vi "LS-335_Hardware_Module.vi"(5 "Enable":bool=TRUE, 6 "PID Settings":T2={"Heater Output (1:1)"=1, "Gain (P) (50.0)"=50.0, "Reset (I) (20.0)"=20.0, "Rate (D) (0.0 %)"=0.0, "Range (0:Off)"=0, "Manual Output (0.00 %)"=0.0} {"Heater Output (1:1)" items=["1"=1, "2"=2]; "Range (0:Off)" items=["Off", "Low (On)", "Medium", "High"]; "Manual Output (0.00 %)" format="%.2f"; "Rate (D) (0.0 %)" format="%.1f"; "Reset (I) (20.0)" format="%.1f"; "Gain (P) (50.0)" format="%.1f"}, 7 "Command":T3, 8 "error in (no error)":errorcluster, 9 "Ramp Rate (0.0)":dbl format="%.1f", 10 "Setpoint (0.0000)":dbl format="%.4f", 11 "VISA resource name":refnum<visa-resource-name>="GPIB0::5::INSTR") -> (0 "error out":errorcluster, 1 "Sensor Data":dbl format="%.4f", 2 "Setpoint":dbl format="%.4f", 3 "Output Value":dbl format="%.1f")   [LabVIEW 2017]
uses:
  LS-335_Hardware_Module Control.ctl
  LS-335 SET PID.ctl
  <instrlib>/Lake Shore 335/Public/Data/Sensor Data (Single Reading).vi
  <instrlib>/Lake Shore 335/Lake Shore 335.lvlib
panel:
  out "Heater Output (1:1)":u16(ring)=1 items=["1"=1, "2"=2]
  out "Power Up Enable (F: Off)":bool
  out "Heater Resistance (1:25 Ohm)":u16(ring)=1 items=["25 Ohm"=1, "50 Ohm"=2]
  out "Input (0:None)":u16(ring)=1 items=["None", "A", "B"]
  out "Mode (0:Off)":u16(ring) items=["Off", "Closed Loop PID", "Zone", "Open Loop", "Monitor Out", "Warmup Supply"]
  out "Max Current (0:User Specified)":u16(ring) items=["User Specified", "0.707 A", "1.0 A", "1.141 A", "1.732 A"]
  out "Max User Current (1.732)":dbl=1.732 format="%.3f"
  out "Heater Out Display (1:Current)":u16(ring)=1 items=["Current"=1, "Power"=2]
  out "Polarity (0:Unipolar)":u16(ring) items=["Unipolar", "Bipolar"]
  out "Output Type (0:Current)":u16(ring) items=["Current", "Voltage"]
  out "Data Source (0:Kelvin)":u16(ring) items=["Kelvin", "Celsius", "Sensor Units"]
  out "Input (0:A)":u16(ring) items=["A", "B"]
  in  "Serial Configuration":T1={"Baud Rate"=57600, "Parity"=1, "Data Bits"=7, "Stop Bits"=10, "Flow Control"=0} {"Flow Control" items=["None", "XON/XOFF", "RTS/CTS", "XON/XOFF & RTS/CTS", "DTR/DSR", "XON/XOFF & DTR/DSR"]; "Stop Bits" items=["1.0"=10, "1.5"=15, "2.0"=20]; "Data Bits" items=["7"=7, "8"=8]; "Parity" items=["None", "Odd", "Even", "Mark", "Space"]; "Baud Rate" items=["300"=300, "600"=600, "1200"=1200, "2400"=2400, "4800"=4800, "9600"=9600, "19200"=19200, "38400"=38400, "57600"=57600]}
  # "LAKE SHORE MODEL 335"
  # "INTERNAL VI SETTINGS. No accesibles desde fuera"
  # "Settings for Either Heater Output"
  # "Settings for Heater Output 2 Only"
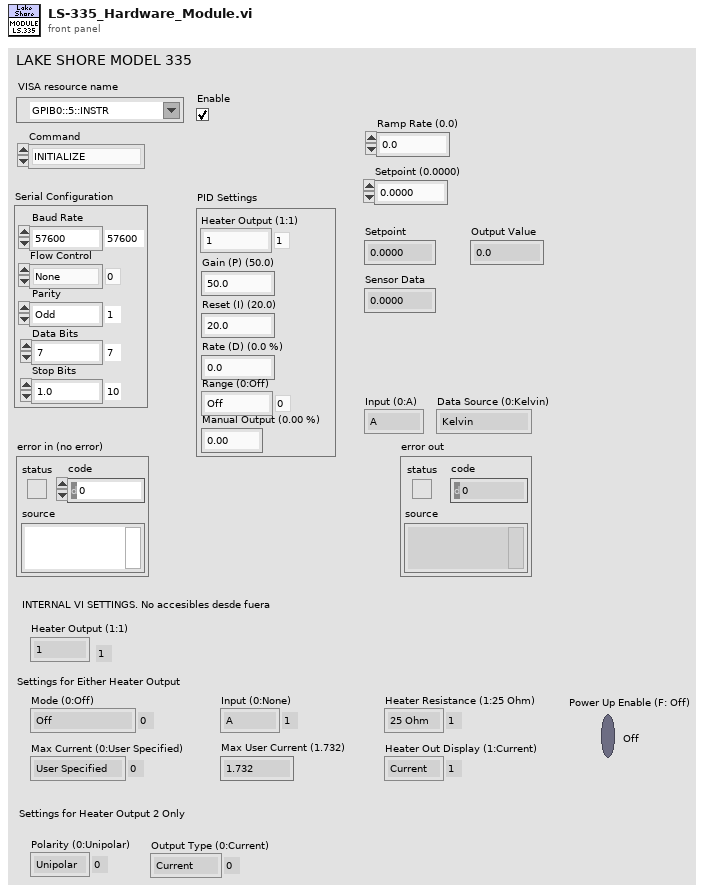
[diagram p1: front panel]
types:
  T1 = cluster{"Baud Rate":u32, "Parity":u16, "Data Bits":u16, "Stop Bits":u16, "Flow Control":u16}
  T2 = typedef "LS-335 SET PID.ctl" = cluster{"Heater Output (1:1)":u16, "Gain (P) (50.0)":dbl, "Reset (I) (20.0)":dbl, "Rate (D) (0.0 %)":dbl, "Range (0:Off)":u16, "Manual Output (0.00 %)":dbl}
  T3 = typedef "LS-335_Hardware_Module Control.ctl" = enum16{"INITIALIZE", "READ TEMPERATURE", "READ CONTROL DATA", "WRITE SETPOINT AND RATE", "WRITE PID AND POWER RANGE", "WRITE CONTROL PARAMETERS", "WRITE INPUT PARAMETERS", "SHUTDOWN"}
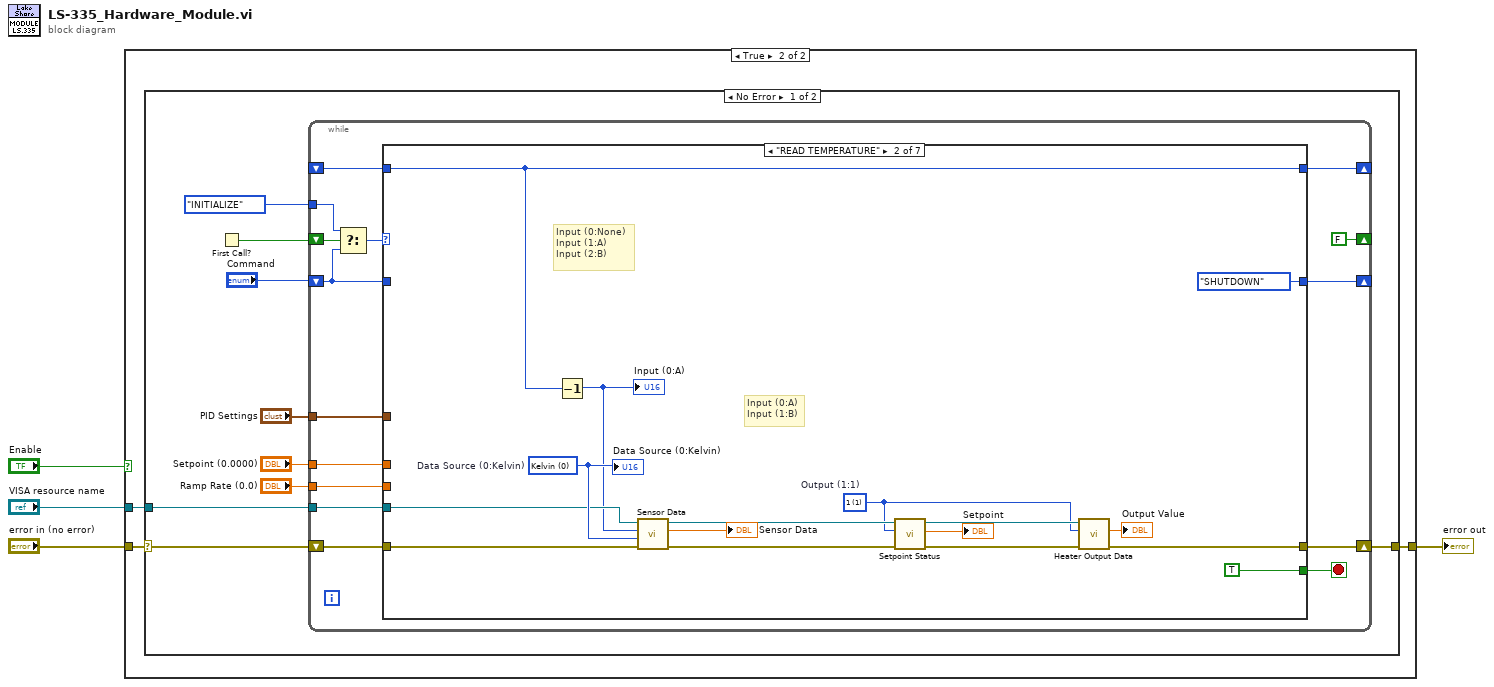
[diagram p0: block diagram]
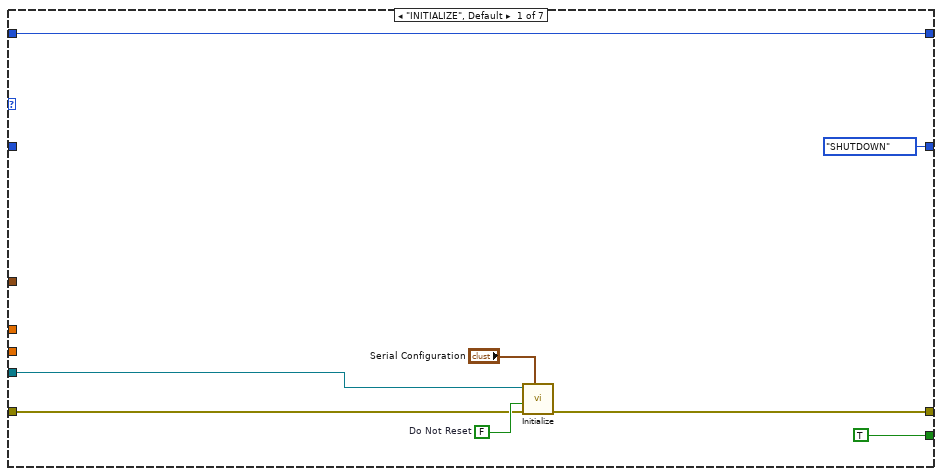
[diagram p3: hidden frame]
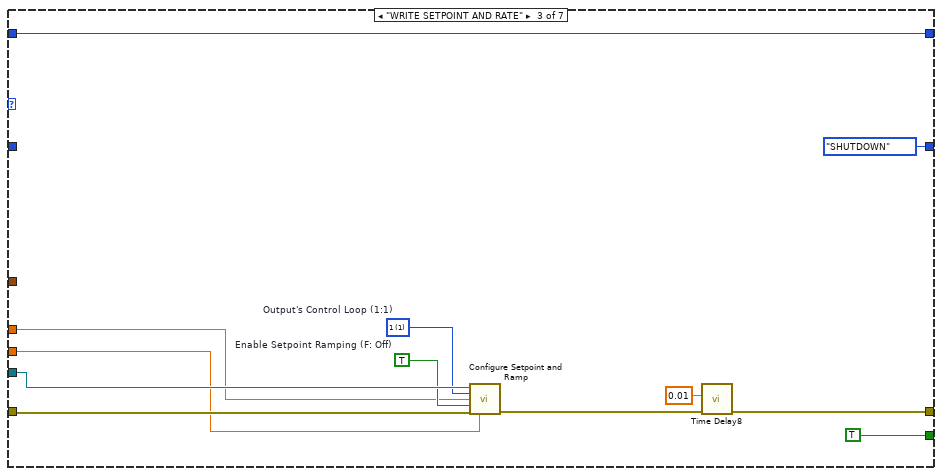
[diagram p4: hidden frame]
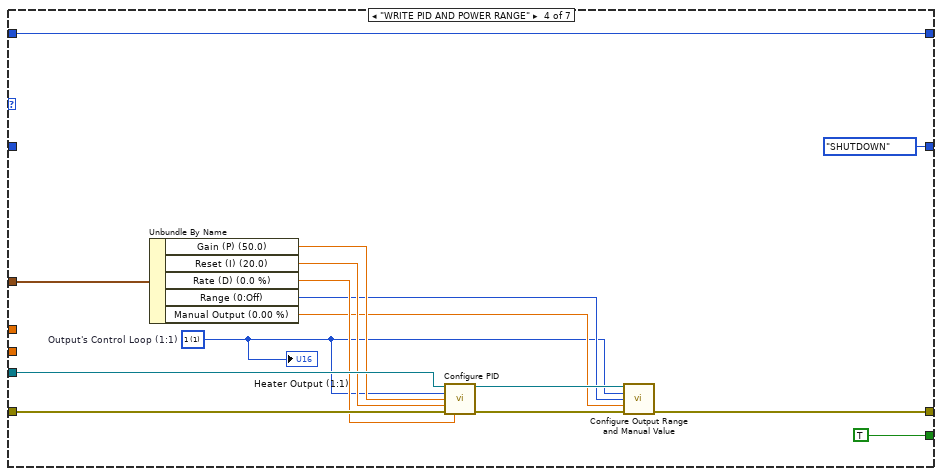
[diagram p5: hidden frame]
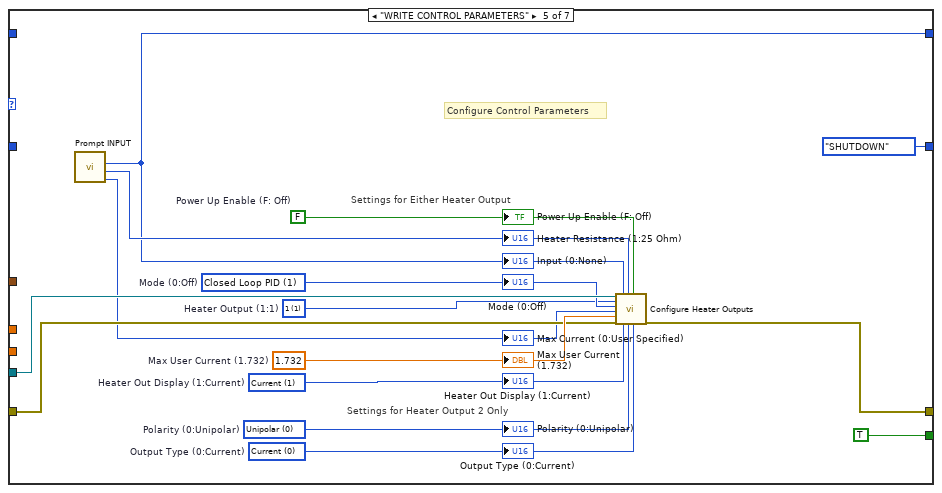
[diagram p6: hidden frame]
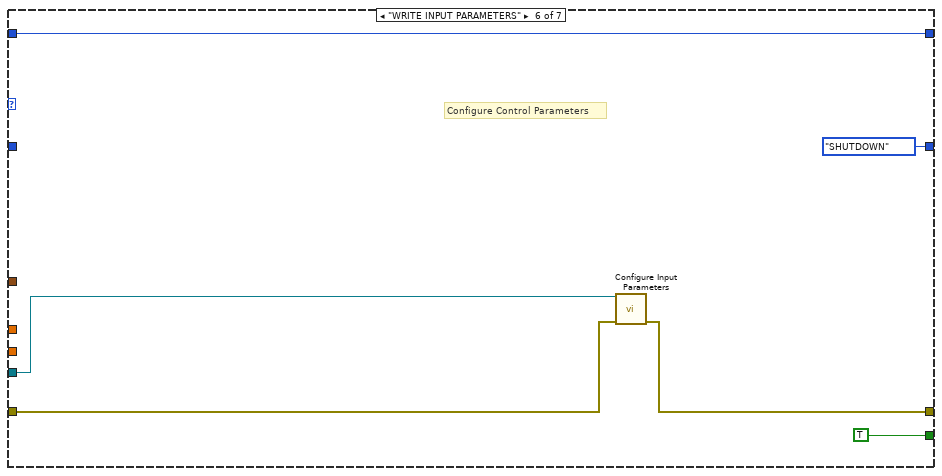
[diagram p7: hidden frame]
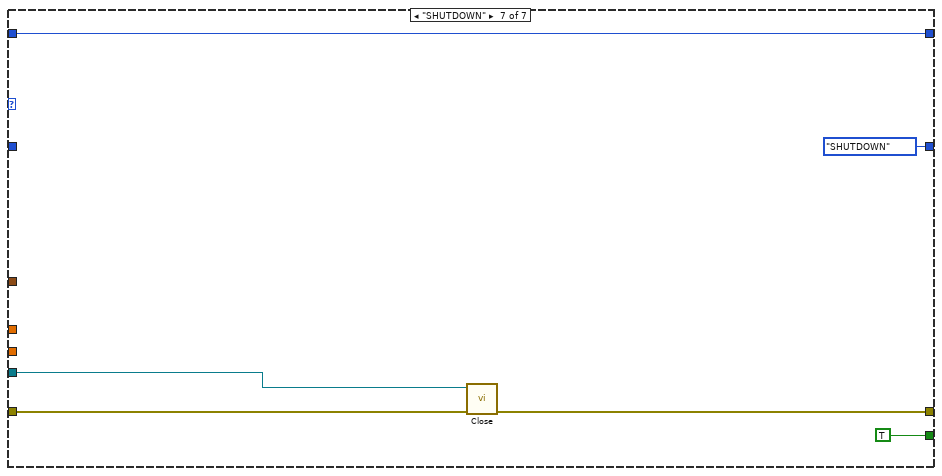
[diagram p8: hidden frame]
diagram:
  n1 = case shown="True" "Enable" {
    tunnel: "error in (no error)" -> [w5 w8]
    tunnel: [w5 w7] -> w3
    tunnel: "VISA resource name" -> [_ w6]
    frame False {
    }
    frame True {
      n2 = case shown="No Error" w8 {
        selector: w8 -> [w15 w111]
        tunnel: [w14 w111] -> w7
        tunnel: w6 -> [w12 _]
        frame No Error {
          n3 = First Call?() -> (First Call?: T/F=w17:bool)
          n4 = while {
            shift-right: [w27] -> _
            shift-left: "Command" -> [w28]
            shift-right: [w25] -> w14
            shift-left: w15 -> [w24]
            shift-right: [FALSE ("First Call?: T/F")] -> _
            shift-left: w17 -> [w32]
            tunnel: LS-335_Hardware_Module_Control."INITIALIZE" ("t") -> [w31]
            tunnel: w12 -> [w23]
            tunnel: "Setpoint (0.0000)" -> [w22]
            tunnel: "Ramp Rate (0.0)" -> [w21]
            tunnel: "PID Settings" -> [w20]
            shift-right: [w19] -> _
            shift-left: _ -> [w18]
            stop <- w26 stop-if-true
            n5 = Select(t=w31, s=w32, f=w28) -> (s? t:f=w29:T3)
            n6 = case shown="\"READ TEMPERATURE\"" w29 {
              tunnel: w28 -> [_ _ _ _ _ _ _]
              tunnel: [LS-335_Hardware_Module_Control."SHUTDOWN" ("s? t:f") LS-335_Hardware_Module_Control."SHUTDOWN" ("s? t:f") LS-335_Hardware_Module_Control."SHUTDOWN" ("s? t:f") LS-335_Hardware_Module_Control."SHUTDOWN" ("s? t:f") LS-335_Hardware_Module_Control."SHUTDOWN" ("s? t:f") LS-335_Hardware_Module_Control."SHUTDOWN" ("s? t:f") LS-335_Hardware_Module_Control."SHUTDOWN" ("s? t:f")] -> w27
              tunnel: [TRUE ("First Call?: T/F") TRUE ("First Call?: T/F") TRUE ("First Call?: T/F") TRUE ("First Call?: T/F") TRUE ("First Call?: T/F") TRUE ("First Call?: T/F") TRUE ("First Call?: T/F")] -> w26
              tunnel: [w36 w44 w66 w75 w90 w103 w108] -> w25
              tunnel: w24 -> [w37 w53 w65 w81 w91 w100 w107]
              tunnel: w23 -> [w35 w54 w63 w82 w92 w101 w109]
              tunnel: w22 -> [_ _ w60 _ _ _ _]
              tunnel: w21 -> [_ _ w59 _ _ _ _]
              tunnel: w20 -> [_ _ _ w71 _ _ _]
              tunnel: [w33 w42 w57 w69 w84 w99 w105] -> w19
              tunnel: w18 -> [w33 w42 w57 w69 _ w99 w105]
              frame "INITIALIZE", Default {
                w38 = FALSE  # Do Not Reset
                n7 = call <instrlib>:"Initialize.vi"("Serial Configuration"="Serial Configuration", "error in (no error)"=w37, "Reset (True)"=w38, "VISA resource name"=w35) -> ("error out"=w36:errorcluster)  [unwired: 6 in, 1 out]
              }
              frame "READ TEMPERATURE" {
                w46 = u16 1 items=["1"=1, "2"=2]  # Output (1:1)
                w55 = u16 0 items=["Kelvin", "Celsius", "Sensor Units"]  # Data Source (0:Kelvin)
                # "Input (0:A)\nInput (1:B)"
                # "Input (0:None)\nInput (1:A)\nInput (2:B)"
                n8 = Decrement(x=w42) -> (x-1=w41:u16)
                "Input (0:A)" <- w41
                n9 = call-poly <instrlib>:"Sensor Data.vi"("error in (no error)"=w53, "Data Source (0:Kelvin)"=w55, "Input (0:A)"=w41, "VISA resource name"=w54) -> ("error out"=w49:errorcluster, "Sensor Data"=→"Sensor Data":dbl, "VISA resource name out"=w50:refnum<visa-resource-name>)  [unwired: 5 in]
                n10 = call <instrlib>:"Setpoint Status.vi"("error in (no error)"=w49, "Output (1:1)"=w46, "VISA resource name"=w50) -> ("error out"=w45:errorcluster, "Setpoint"=→"Setpoint":dbl, "VISA resource name out"=w47:refnum<visa-resource-name>)  [unwired: 6 in]
                n11 = call <instrlib>:"Heater Output Data.vi"("error in (no error)"=w45, "Heater Output (1:1)"=w46, "VISA resource name"=w47) -> ("error out"=w44:errorcluster, "Output Value"=→"Output Value":dbl)  [unwired: 6 in, 1 out]
                "Data Source (0:Kelvin)" <- w55
              }
              frame "WRITE SETPOINT AND RATE" {
                w61 = TRUE  # Enable Setpoint Ramping (F: Off)
                w62 = u16 1 items=["1"=1, "2"=2]  # Output's Control Loop (1:1)
                n12 = call <instrlib>:"Configure Setpoint and Ramp.vi"("VISA resource name"=w63, "Output's Control Loop (1:1)"=w62, "Setpoint (0.0000)"=w60, "Enable Setpoint Ramping (F: Off)"=w61, "error in (no error)"=w65, "Ramp Rate (0.0)"=w59) -> ("error out"=w64:errorcluster)  [unwired: 8 in, 1 out]
                n13 = call "Time Delay8"("error in (no error)"=w64, "Delay Time (s)"=0.01) -> ("error out"=w66:errorcluster)  [unwired: 9 in]
              }
              frame "WRITE PID AND POWER RANGE" {
                w70 = u16 1 items=["1"=1, "2"=2]  # Output's Control Loop (1:1)
                n14 = Unbundle By Name(w71) -> ("Gain (P) (50.0)"=w80:dbl, "Reset (I) (20.0)"=w79:dbl, "Rate (D) (0.0 %)"=w78:dbl, "Range (0:Off)"=w73:u16, "Manual Output (0.00 %)"=w74:dbl)
                n15 = call <instrlib>:"Configure PID.vi"("VISA resource name"=w82, "Output's Control Loop (1:1)"=w70, "Gain (P) (50.0)"=w80, "Reset (I) (20.0)"=w79, "error in (no error)"=w81, "Rate (D) (0.0 %)"=w78) -> ("VISA resource name out"=w77:refnum<visa-resource-name>, "error out"=w76:errorcluster)  [unwired: 8 in]
                n16 = call <instrlib>:"Configure Output Range and Manual Value.vi"("VISA resource name"=w77, "Heater Output (1:1)"=w70, "Range (0:Off)"=w73, "Manual Output (0.00 %)"=w74, "error in (no error)"=w76) -> ("error out"=w75:errorcluster)  [unwired: 9 in, 1 out]
                "Heater Output (1:1)" <- w70
              }
              frame "WRITE CONTROL PARAMETERS" {
                w87 = u16 1 items=["1"=1, "2"=2]  # Heater Output (1:1)
                w94 = 1.732  # Max User Current (1.732)
                w95 = u16 1 items=["Current"=1, "Power"=2]  # Heater Out Display (1:Current)
                w96 = u16 0 items=["Unipolar", "Bipolar"]  # Polarity (0:Unipolar)
                w97 = u16 0 items=["Current", "Voltage"]  # Output Type (0:Current)
                w93 = FALSE  # Power Up Enable (F: Off)
                w88 = u16 1 items=["Off", "Closed Loop PID", "Zone", "Open Loop", "Monitor Out", "Warmup Supply"]  # Mode (0:Off)
                # "Settings for Either Heater Output"
                # "Settings for Heater Output 2 Only"
                # "Configure Control Parameters"
                n17 = call "Prompt INPUT.vi"() -> ("Max Current (0:User Specified)"=w85:u16, "Heater Resistance (1:25 Ohm)"=w86:u16, "Input (0:None)"=w84:u16)  [unwired: 8 in, 1 out]
                "Heater Resistance (1:25 Ohm)" <- w86
                "Input (0:None)" <- w84
                "Max Current (0:User Specified)" <- w85
                n18 = call <instrlib>:"Configure Heater Outputs.vi"("VISA resource name"=w92, "Heater Output (1:1)"=w87, "Mode (0:Off)"=w88, "Max Current (0:User Specified)"=w85, "Max User Current (1.732)"=w94, "error in (no error)"=w91, "Input (0:None)"=w84, "Heater Out Display (1:Current)"=w95, "Heater Resistance (1:25 Ohm)"=w86, "Polarity (0:Unipolar)"=w96, "Power Up Enable (F: Off)"=w93, "Output Type (0:Current)"=w97) -> ("error out"=w90:errorcluster)  [unwired: 6 in, 1 out]
                "Power Up Enable (F: Off)" <- w93
                "Mode (0:Off)" <- w88
                "Max User Current (1.732)" <- w94
                "Heater Out Display (1:Current)" <- w95
                "Polarity (0:Unipolar)" <- w96
                "Output Type (0:Current)" <- w97
              }
              frame "WRITE INPUT PARAMETERS" {
                # "Configure Control Parameters"
                n19 = call <instrlib>:"Configure Input Parameters.vi"("VISA resource name"=w101, "error in (no error)"=w100) -> ("error out"=w103:errorcluster)  [unwired: 12 in, 1 out]
              }
              frame "SHUTDOWN" {
                n20 = call <instrlib>:"Close.vi"("error in (no error)"=w107, "VISA resource name"=w109) -> ("error out"=w108:errorcluster)  [unwired: 9 in]
              }
            }
          }
        }
        frame Error {
        }
      }
    }
  }
  "error out" <- w3
